vi "composePotentialFieldVelocities.vi"(9 "multiplier":dbl, 10 "potentialFieldVelocities":dbl[](array[numeric]), 11 "Robot in":refnum<class "Robot.lvclass">) -> (3 "v_tang/v_norm":dbl[](array[numeric]))   [LabVIEW 2020, in "Robot.lvclass"]
uses:
  Robot.lvclass
  Robot.lvclass/Robot.ctl
  <vilib>/Analysis/coordinate.llb/2D Cartesian Coordinate Rotation (Scalar).vi
  Read v_tang.vi
  Read v_norm.vi
  Read orientation.vi
  <vilib>/Analysis/NI_AALPro.lvlib
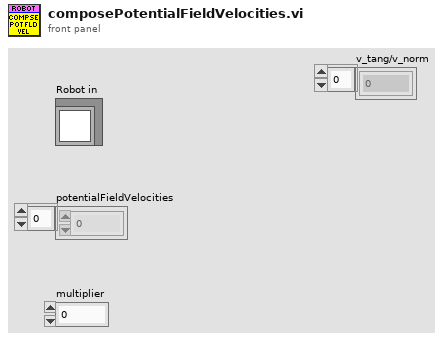
[diagram p1: front panel]
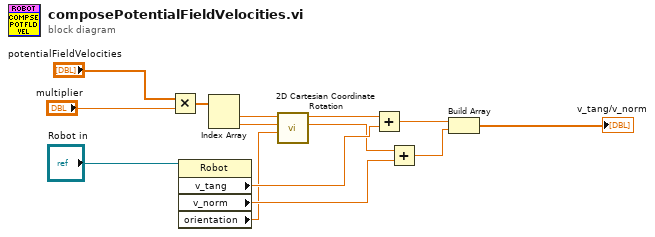
[diagram p0: block diagram]
diagram:
  n1 = Multiply(x="potentialFieldVelocities", y="multiplier") -> (x*y=w6:dbl[])
  n2 = property class="Robot"(reference="Robot in") -> ("v_tang"=w12:dbl, "v_norm"=w10:dbl, "orientation"=w7:dbl)  [unwired: 1 in, 2 out]
  n3 = Index Array(array=w6) -> (element #1=w8:dbl, element #2=w4:dbl)  [unwired: 2 in]
  n4 = call-poly <vilib>:"2D Cartesian Coordinate Rotation.vi"("theta"=w7, "y"=w4, "x"=w8) -> ("y out"=w9:dbl, "x out"=w11:dbl)  [unwired: 6 in, 1 out]
  n5 = Add(x=w11, y=w12) -> (x+y=w3:dbl)
  n6 = Add(x=w9, y=w10) -> (x+y=w2:dbl)
  n7 = Build Array(w3, w2) -> (→"v_tang/v_norm":dbl[])
